vi "Motion@Go(SingleAxis)__Parameter.vi"(1 "ParamterIn":string) -> (0 "ParamterOut":string)   [LabVIEW 2019]
panel:
  in  "Position":string(combo)
  in  "Speed":string(combo)
  in  "Axis":string(combo)
  in  "MotorName":string(combo)
  in  "Confirm":bool
  # "Motor@Go $Motor,$Axis,$Speed,$X(,$Y,$Z,$U...)"
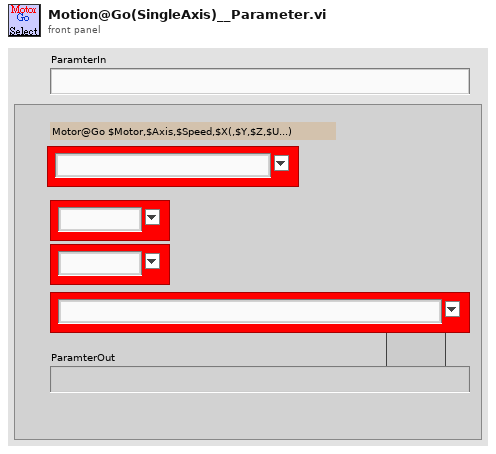
[diagram p1: front panel]
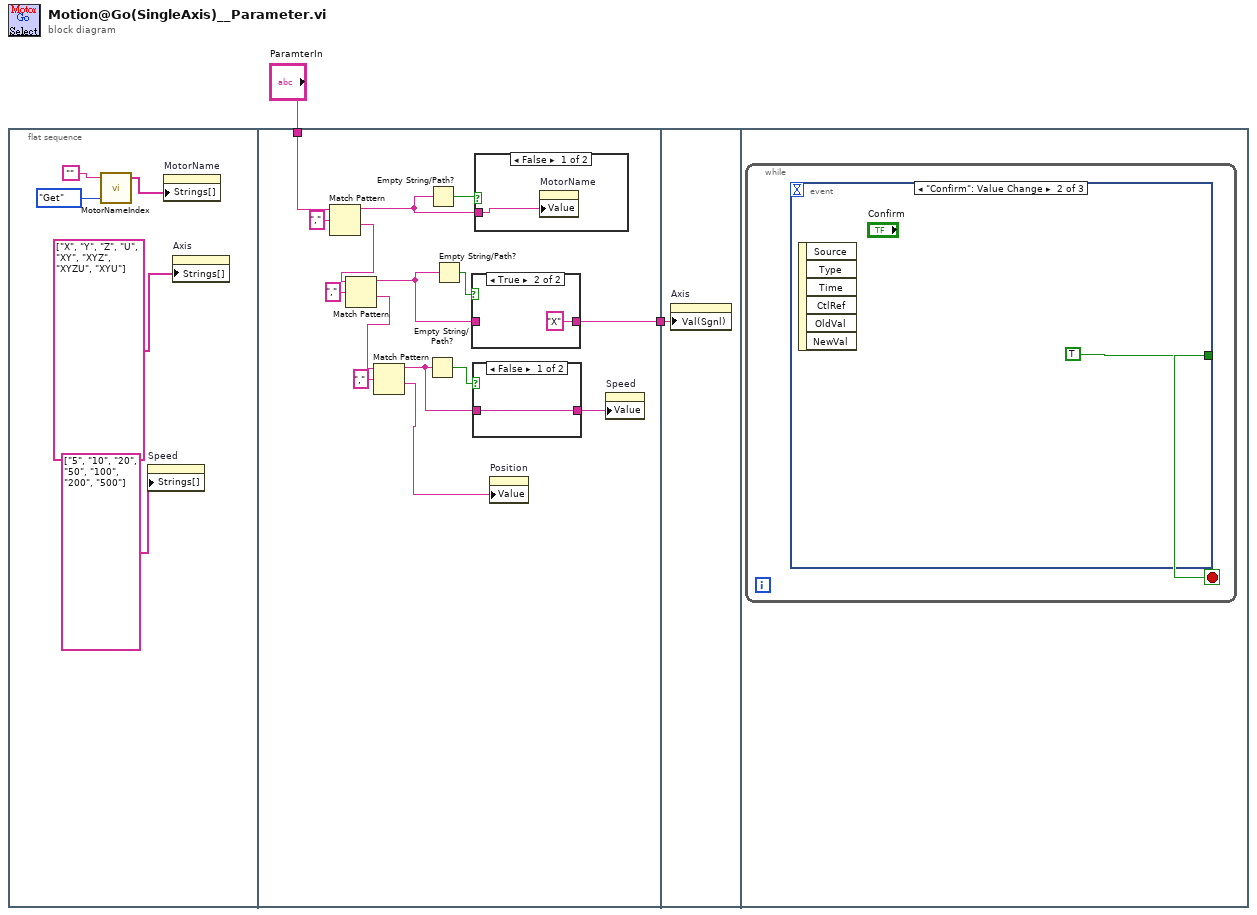
[diagram p0: block diagram]
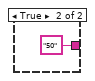
[diagram p2: hidden frame]
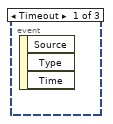
[diagram p5: hidden frame]
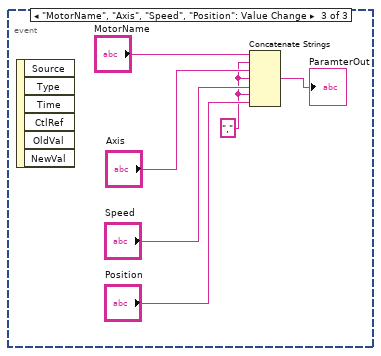
[diagram p6: hidden frame]
diagram:
  n1 = flat-sequence {
    tunnel: "ParamterIn" -> [w19]
    tunnel: [w20] -> w1
    tunnel: w1 -> [w28]
    frame #0 {
      n2 = call "MotorNameIndex.vi"("OP"=enum16{"Get", "Update", "Init"}."Get", "MotorName"="") -> ("MotorList"=w5:string[])  [unwired: 1 in, 2 out]
      n3 = property on="Speed" class="CmbBox"("Strings[]"=string[] ["5", "10", "20", "50", "100", "200", "500"] ("Strings []")) -> ()  [unwired: 2 in, 2 out]
      n4 = property on="MotorName" class="CmbBox"("Strings[]"=w5) -> ()  [unwired: 2 in, 2 out]
      n5 = property on="Axis" class="CmbBox"("Strings[]"=string[] ["X", "Y", "Z", "U", "XY", "XYZ", "XYZU", "XYU"] ("Strings []")) -> ()  [unwired: 2 in, 2 out]
    }
    frame #1 {
      n6 = Match Pattern(string=w19, regular expression="," ("search string")) -> (before substring=w17:string, after substring=w15:string)  [unwired: 1 in, 2 out]
      n7 = Match Pattern(string=w15, regular expression="," ("search string")) -> (before substring=w14:string, after substring=w12:string)  [unwired: 1 in, 2 out]
      n8 = Match Pattern(string=w12, regular expression="," ("search string")) -> (before substring=w8:string, after substring=w9:string)  [unwired: 1 in, 2 out]
      n9 = Empty String/Path?(string/path=w8) -> (empty?=w11:bool)
      n10 = Empty String/Path?(string/path=w17) -> (empty?=w22:bool)
      n11 = Empty String/Path?(string/path=w14) -> (empty?=w21:bool)
      n12 = case shown="True" w21 {
        tunnel: [w25 "X" ("ParamterIn")] -> w20
        tunnel: w14 -> [w25 _]
        frame False {
        }
        frame True {
        }
      }
      n13 = case shown="False" w11 {
        tunnel: [w23 "50" ("ParamterIn")] -> w10
        tunnel: w8 -> [w23 _]
        frame False {
        }
        frame True {
        }
      }
      n14 = case shown="False" w22 {
        tunnel: w17 -> [w27 _]
        frame False {
          n15 = property on="MotorName" class="CmbBox"("Value"=w27) -> ()  [unwired: 2 in, 2 out]
        }
        frame True {
        }
      }
      n16 = property on="Position" class="CmbBox"("Value"=w9) -> ()  [unwired: 2 in, 2 out]
      n17 = property on="Speed" class="CmbBox"("Value"=w10) -> ()  [unwired: 2 in, 2 out]
    }
    frame #2 {
      n18 = property on="Axis" class="CmbBox"("Val(Sgnl)"=w28) -> ()  [unwired: 2 in, 2 out]
    }
    frame #3 {
      n19 = while {
        stop <- w29 stop-if-true
        n20 = event shown="[1] \"Confirm\": Value Change" {
          selector: _ -> [_ _ _]
          dyn-events: _ -> [_ _ _]
          timeout: _ -> [_ _ _]
          tunnel: [_ TRUE _] -> w29
          event Timeout {
            n21 = event-data() -> ()  [unwired: 1 in, 3 out]
          }
          event "Confirm": Value Change {
            n22 = event-data() -> ()  [unwired: 1 in, 6 out]
          }
          event "MotorName", "Axis", "Speed", "Position": Value Change {
            w31 = "," ("string")
            n23 = event-data() -> ()  [unwired: 1 in, 6 out]
            n24 = Concatenate Strings("MotorName", w31, "Axis", w31, "Speed", w31, "Position") -> (→"ParamterOut":string)
          }
        }
      }
    }
  }
